vi "ReadFile.vi"(8 "error in (no error)":errorcluster, 10 "file":path, 11 "baseParser in":refnum<class "baseParser.lvclass">) -> (0 "error out":errorcluster, 3 "baseParser out":refnum<class "baseParser.lvclass">)   [LabVIEW 2013, in "baseParser.lvclass"]
uses:
  baseParser.lvclass
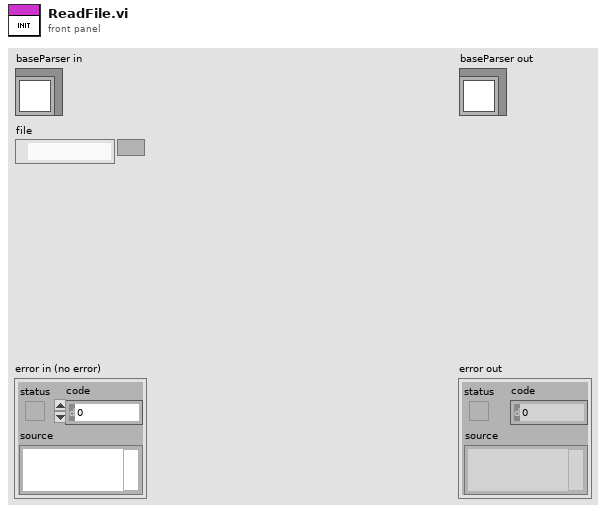
[diagram p1: front panel]
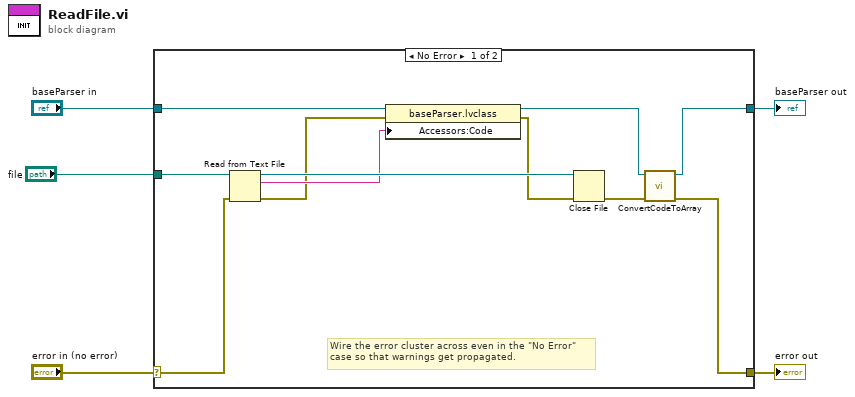
[diagram p0: block diagram]
diagram:
  n1 = case shown="No Error" "error in (no error)" {
    selector: "error in (no error)" -> [w10 w18]
    tunnel: [w6 w18] -> w4
    tunnel: [w8 w17] -> w2
    tunnel: "baseParser in" -> [w16 w17]
    tunnel: "file" -> [w14 _]
    frame No Error {
      # "Wire the error cluster across even in the \"No Error\"\ncase so that warnings get propagated."
      n2 = Read from Text File(file (use dialog)=w14, error in=w10) -> (refnum out=w15:refnum<file>, text=w13:string, error out=w12:errorcluster)  [unwired: 2 in, 1 out]
      n3 = property class="baseParser.lvclass"(reference=w16, error in=w12, "Accessors:Code"=w13) -> (reference out=w9:refnum<class "baseParser.lvclass">, error out=w11:errorcluster)
      n4 = Close File(refnum=w15, error in=w11) -> (error out=w7:errorcluster)  [unwired: 1 out]
      n5 = call "ConvertCodeToArray.vi"("error in (no error)"=w7, "baseParser in"=w9) -> ("error out"=w6:errorcluster, "baseParser out"=w8:refnum<class "baseParser.lvclass">)  [unwired: 8 in]
    }
    frame Error {
    }
  }
  "error out" <- w4
  "baseParser out" <- w2
